vi "testKM1.vi"() -> ()   [LabVIEW 2014]
panel:
  in  "count 2":dbl
  in  "count":dbl
  in  "R":dbl
  in  "s":dbl
  out "Frequency 2":dbl
  out "Sine":dynamicdata(graph)
  in  "stop":bool
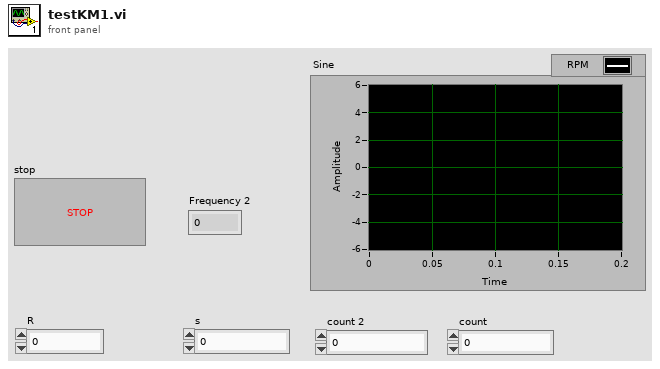
[diagram p1: front panel]
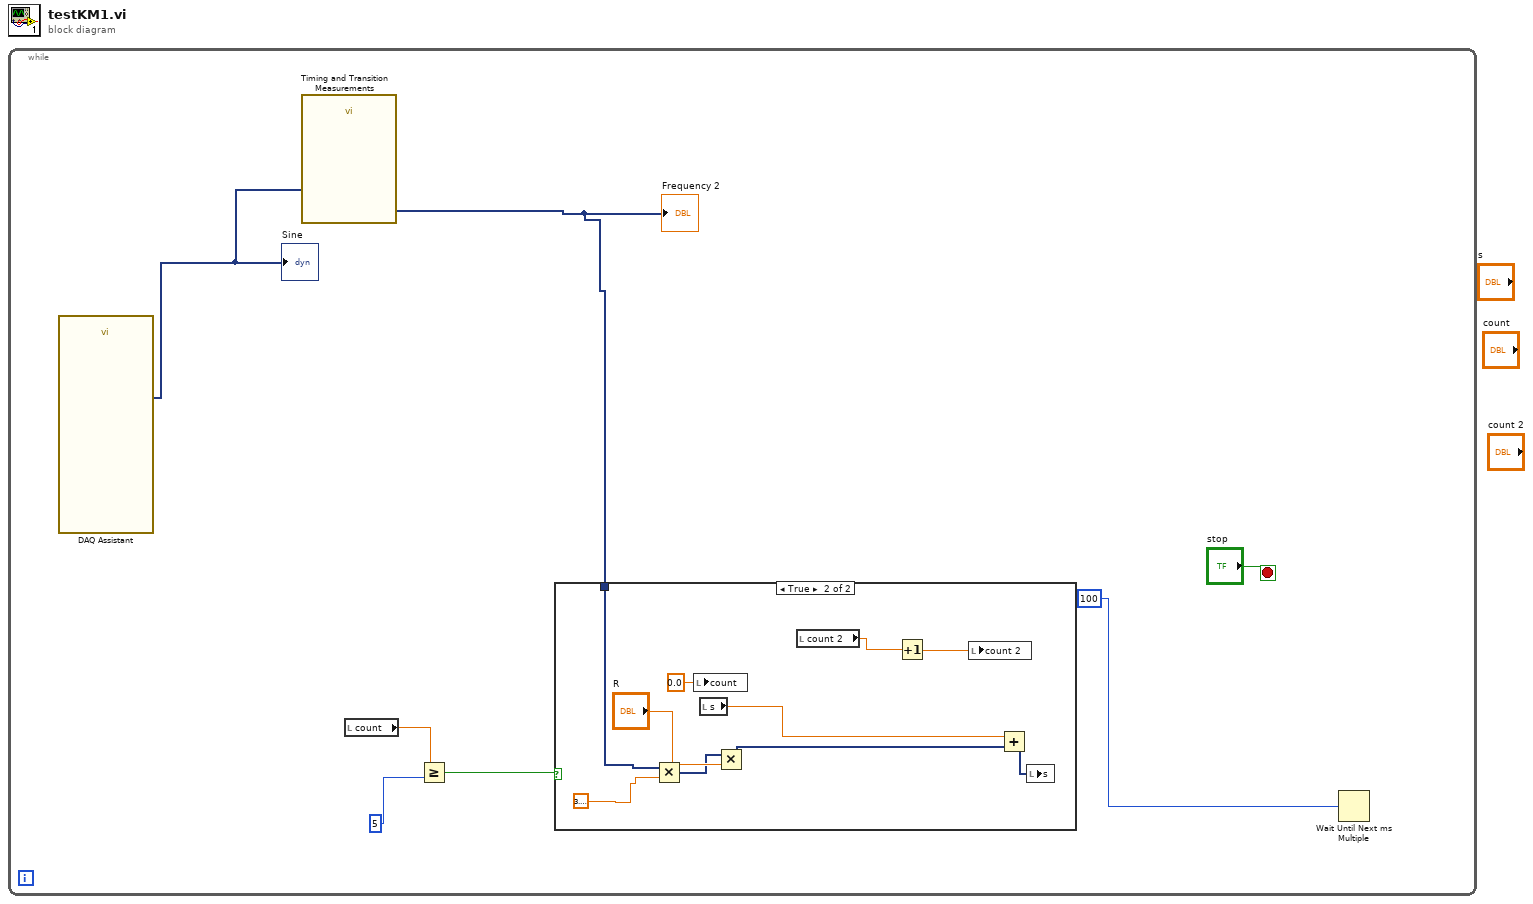
[diagram p0: block diagram]
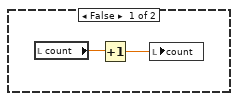
[diagram p2: hidden frame]
diagram:
  n1 = while {
    stop <- "stop" stop-if-true
    n2 = call "DAQ Assistant"() -> ("data"=w1:dynamicdata)  [unwired: 16 in, 3 out]
    "Sine" <- w1
    n3 = call "Timing and Transition Measurements"("Signals"=w1) -> ("Frequency"=w2:dynamicdata)  [unwired: 9 in, 1 out]
    "Frequency 2" <- w2
    n4 = local read "count"() -> (w6:dbl)
    n5 = Greater Or Equal?(x=w6, y=5) -> (x >= y?=w4:bool)
    n6 = case shown="True" w4 {
      tunnel: w2 -> [_ w17]
      frame False {
        n7 = local read "count"() -> (w9:dbl)
        n8 = Increment(x=w9) -> (x+1=w8:dbl)
        n9 = local write "count"(w8) -> ()
      }
      frame True {
        n10 = Multiply(x=w17, y=3.141592653589793) -> (x*y=w18:dynamicdata)
        n11 = local write "count"(0.0 ("count")) -> ()
        n12 = local read "s"() -> (w14:dbl)
        n13 = Multiply(x=w18, y="R") -> (x*y=w15:dynamicdata)
        n14 = local read "count 2"() -> (w11:dbl)
        n15 = Increment(x=w11) -> (x+1=w10:dbl)
        n16 = local write "count 2"(w10) -> ()
        n17 = Add(x=w14, y=w15) -> (x+y=w13:dynamicdata)
        n18 = local write "s"(w13) -> ()
      }
    }
    n19 = Wait Until Next ms Multiple(millisecond multiple=u32 100) -> ()  [unwired: 1 out]
  }
